vi "FTW-Producer-Enqueue.vi"(0 "FTW-Producer In":refnum<class "FTW-Producer.lvclass">, 5 "Header":string, 7 "Body":string, 9 "Timeout":i32=1000 format="%dmsec", 11 "error in":errorcluster) -> (4 "FTW-Producer Out":refnum<class "FTW-Producer.lvclass">, 10 "Timed out?":bool, 14 "Send Time":dbl format="%.6fsec", 15 "error out":errorcluster)   [LabVIEW 2013, in "FTW-Producer.lvclass"]
uses:
  FTW-Producer.lvclass
  FTW-Producer.lvclass/FTW-Producer.ctl
  Endpoint/FTW-Endpoint.lvclass
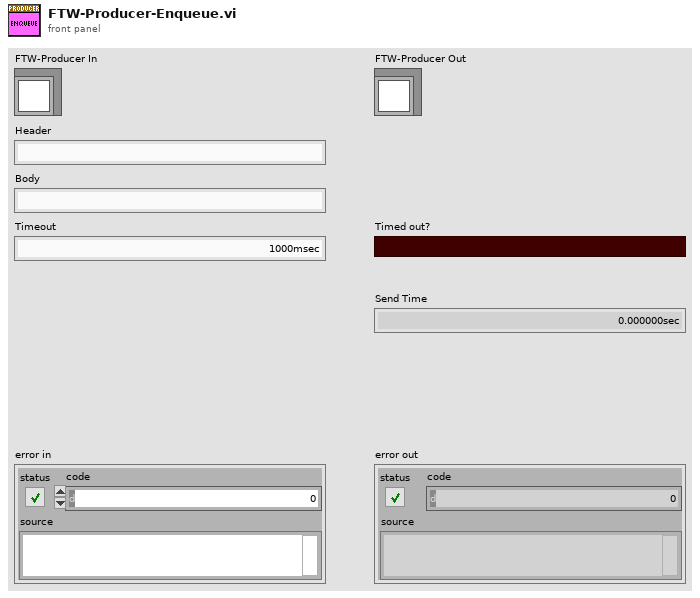
[diagram p1: front panel]
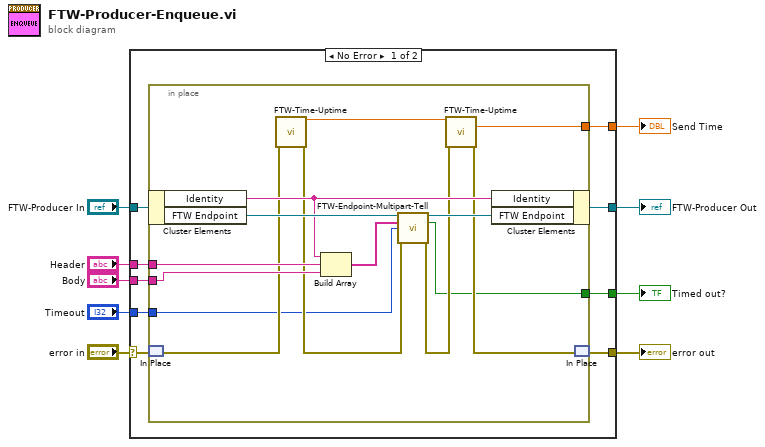
[diagram p0: block diagram]
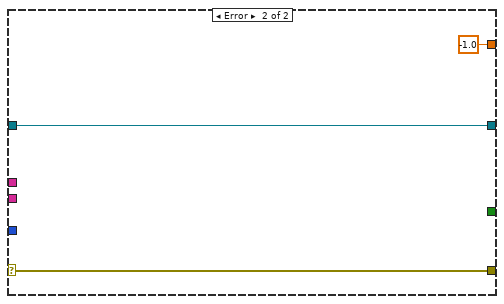
[diagram p2: hidden frame]
diagram:
  n1 = case shown="No Error" "error in" {
    selector: "error in" -> [w16 w35]
    tunnel: [w15 w35] -> w6
    tunnel: [w17 w34] -> w8
    tunnel: "FTW-Producer In" -> [w18 w34]
    tunnel: "Header" -> [w14 _]
    tunnel: "Body" -> [w13 _]
    tunnel: "Timeout" -> [w12 _]
    tunnel: [w11 _] -> w2
    tunnel: [w10 -1.0 ("Elapsed Time")] -> w1
    frame No Error {
      n2 = in-place {
        in-place-border: w14 -> [w30]
        in-place-border: w13 -> [w29]
        in-place-border: w12 -> [w21]
        in-place-border: [w19] -> w11
        in-place-border: [w26] -> w10
        n3 = in-place-cluster #1(w18) -> ("Identity"=w28:string, "FTW Endpoint"=w32:refnum<class "FTW-Endpoint.lvclass">)
        n4 = in-place-match #2(w16) -> (w25:errorcluster)
        n5 = call "FTW-Time-Uptime.vi"("error in"=w25) -> ("Current Uptime"=w22:dbl, "error out"=w24:errorcluster)  [unwired: 12 in, 1 out]
        n6 = Build Array(w28, w30, w29) -> (w27:string[])
        n7 = call-dynamic "FTW-Endpoint-Multipart-Tell.vi"("FTW Endpoint"=w32, "Multipart Message"=w27, "Timeout"=w21, "error in"=w24) -> ("FTW Endpoint out"=w31:refnum<class "FTW-Endpoint.lvclass">, "Timed out?"=w19:bool, "error out"=w20:errorcluster)  [unwired: 9 in]
        n8 = call "FTW-Time-Uptime.vi"("Previous Uptime"=w22, "error in"=w20) -> ("Elapsed Time"=w26:dbl, "error out"=w23:errorcluster)  [unwired: 11 in, 1 out]
        n9 = in-place-cluster #1("Identity"=w28, "FTW Endpoint"=w31) -> (w17:refnum<class "FTW-Producer.lvclass">)
        n10 = in-place-match #2(w23) -> (w15:errorcluster)
      }
    }
    frame Error {
    }
  }
  "FTW-Producer Out" <- w8
  "error out" <- w6
  "Timed out?" <- w2
  "Send Time" <- w1
